vi "Weighted_Cross_Moments_raw.vi"(0 "AI Cluster 1":T5={"Colour"=0, "Inst type"=enum."Pitot-static tube", "Inst name"="Manometer voltage", "Symbol"="U", "Code name"="", "Extra Info"="U", "Inst Array"=enum."PWA", "Extra Titles"=[], "Extra Values"=[], "U"=0.0, "u^2"=0.0, "u^3"=0.0, "u^4"=0.0, "Skew_u"=0.0, "Kurt_u"=0.0, "Sd Error in Mean"=0.0, "% u'/U"=0.0, "X"=0.0, "Y"=0.0, "Z"=0.0, "Timescale integral Estimate"=0.0, "Sd Error in Variance"=0.0, "Calib File"=path "", "Calib Constants"=[], "Output Position"=FALSE, "Stats"=enum."None", "Av Sampling Rate"=0.0, "Av No of Samples"=0.0, "Total Meas Time (s)"=0.0, "ADAM Ch Name"="", "Max value"=0.0, "Min value"=0.0, "Req Sample Rate Hz"=0.0, "Sync Delay Time (s)"=0.0, "Ch No"=0, "Device"="", "Use Latest Calib"=FALSE, "Port"="", "Metadata Ch Names"=[], "Metadata Ch Values"=[], "Label"=""} {"Sync Delay Time (s)" format="%.4f"; "Total Meas Time (s)" format="%_5g"; "Sd Error in Variance" format="%_3g"; "Skew_u" format="%_3g"; "% u'/U" format="%_3g"; "Sd Error in Mean" format="%_3g"; "Kurt_u" format="%_3g"; "u^4" format="%_3g"; "u^3" format="%_3g"; "U" format="%_3g"; "u^2" format="%_3g"}, 1 "AI Cluster 2":T5={"Colour"=0, "Inst type"=enum."Pitot-static tube", "Inst name"="Manometer voltage", "Symbol"="U", "Code name"="", "Extra Info"="U", "Inst Array"=enum."PWA", "Extra Titles"=[], "Extra Values"=[], "U"=0.0, "u^2"=0.0, "u^3"=0.0, "u^4"=0.0, "Skew_u"=0.0, "Kurt_u"=0.0, "Sd Error in Mean"=0.0, "% u'/U"=0.0, "X"=0.0, "Y"=0.0, "Z"=0.0, "Timescale integral Estimate"=0.0, "Sd Error in Variance"=0.0, "Calib File"=path "", "Calib Constants"=[], "Output Position"=FALSE, "Stats"=enum."None", "Av Sampling Rate"=0.0, "Av No of Samples"=0.0, "Total Meas Time (s)"=0.0, "ADAM Ch Name"="", "Max value"=0.0, "Min value"=0.0, "Req Sample Rate Hz"=0.0, "Sync Delay Time (s)"=0.0, "Ch No"=0, "Device"="", "Use Latest Calib"=FALSE, "Port"="", "Metadata Ch Names"=[], "Metadata Ch Values"=[], "Label"=""} {"Sync Delay Time (s)" format="%.4f"; "Total Meas Time (s)" format="%_5g"; "Sd Error in Variance" format="%_3g"; "Skew_u" format="%_3g"; "% u'/U" format="%_3g"; "Sd Error in Mean" format="%_3g"; "Kurt_u" format="%_3g"; "u^4" format="%_3g"; "u^3" format="%_3g"; "U" format="%_3g"; "u^2" format="%_3g"}, 2 "Time Cluster 1":T3, 3 "Time Cluster 2":T3, 5 "Shift Cluster In":T2 {"Cross Correlation" format="%.2f"; "Stats" format="%.2f"}, 7 "Shift Input":T1, 9 "interp. method":enum16{"nearest", "linear"}(ring)=enum."linear", 10 "Time (s) 1":dbl[](array[numeric]), 11 "Time (s) 2":dbl[](array[numeric])) -> (13 "Shift Output":T1, 17 "output cluster":T4 {"Time Window (ms)" format="%.2f"; "w^2 Paired" format="%.2f"; "u^2 Paired" format="%.2f"; "u^2w^2" format="%.2f"; "u^3w" format="%.2f"; "uw^3" format="%.2f"; "uw/u'w'" format="%.2f"; "uw^2" format="%.2f"; "u^2w" format="%.2f"; "uw" format="%.2f"}, 19 "Shift Cluster Out":T2 {"Cross Correlation" format="%.2f"; "Stats" format="%.2f"})   [LabVIEW 2021]
uses:
  Controls/Analysis_info_cluster.ctl
  Controls/Inst_type.ctl
  Controls/Instrument_Array.ctl
  Controls/Correlation_cluster1.ctl
  Controls/Time_Trace_Cluster.ctl
  Controls/Cross_Moments_Shift_Cluster.ctl
  Controls/Shift_Cluster.ctl
  <vilib>/Analysis/baseanly.llb/Mean (DBL).vi
  Globals/Meas_global.vi
  <vilib>/Analysis/NI_AALBase.lvlib
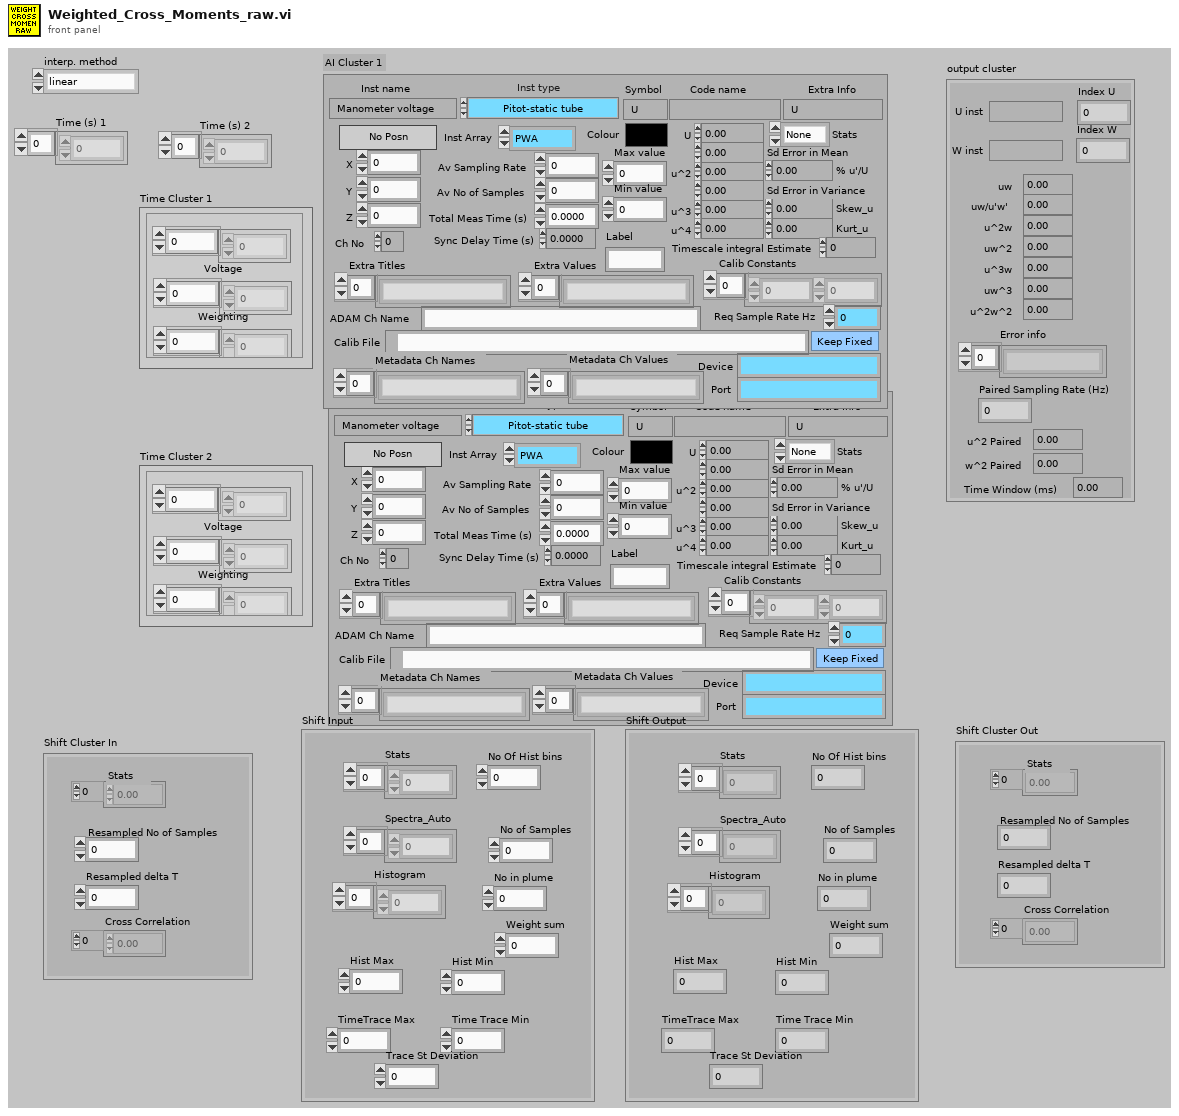
[diagram p1: front panel]
types:
  T1 = typedef "Shift_Cluster.ctl" = cluster{"Stats":dbl[], "Spectra_Auto":dbl[], "Histogram":dbl[], "Hist Max":dbl, "Hist Min":dbl, "No of Samples":i32, "No in plume":i32, "Weight sum":dbl, "No Of Hist bins":i32, "TimeTrace Max":dbl, "Time Trace Min":dbl, "Trace St Deviation":dbl}
  T2 = typedef "Cross_Moments_Shift_Cluster.ctl" = cluster{"Stats":dbl[], "Resampled No of Samples":i32, "Resampled delta T":dbl, "Cross Correlation":dbl[]}
  T3 = typedef "Time_Trace_Cluster.ctl" = cluster{"Weighting":dbl[], "Voltage":dbl[], "Eng Values":dbl[]}
  T4 = typedef "Correlation_cluster1.ctl" = cluster{"U inst":string, "uw":dbl, "u^2w":dbl, "uw^2":dbl, "uw/u'w'":dbl, "W inst":string, "uw^3":dbl, "u^3w":dbl, "u^2w^2":dbl, "Index U":i32, "Index W":i32, "Error info":string[], "Paired Sampling Rate (Hz)":dbl, "u^2 Paired":dbl, "w^2 Paired":dbl, "Time Window (ms)":dbl}
  T5 = typedef "Analysis_info_cluster.ctl" = cluster{"Colour":u32, "Inst type":T6, "Inst name":string, "Symbol":string, "Code name":string, "Extra Info":string, "Inst Array":T7, "Extra Titles":string[], "Extra Values":string[], "U":dbl, "u^2":dbl, "u^3":dbl, "u^4":dbl, "Skew_u":dbl, "Kurt_u":dbl, "Sd Error in Mean":dbl, "% u'/U":dbl, "X":dbl, "Y":dbl, "Z":dbl, "Timescale integral Estimate":dbl, "Sd Error in Variance":dbl, "Calib File":path, "Calib Constants":dbl[], "Output Position":bool, "Stats":enum16{"None", "Basic", "Full"}, "Av Sampling Rate":dbl, "Av No of Samples":dbl, "Total Meas Time (s)":dbl, "ADAM Ch Name":string, "Max value":dbl, "Min value":dbl, "Req Sample Rate Hz":dbl, "Sync Delay Time (s)":dbl, "Ch No":i16, "Device":string, "Use Latest Calib":bool, "Port":string, "Metadata Ch Names":string[], "Metadata Ch Values":string[], "Label":string}
  T6 = typedef "Inst_type.ctl" = enum16{"Raw voltage", "Raw with zero offsetting", "Propeller anemometer", "Pressure Transducer", "Pitot-static tube", "Hot wire", "Cross wire 1", "Cross wire 2", "Generic Linear", "Generic Polynomial", "Generic BackPoly", "Fast FID", "Thermocouple", "Cold wire", "Pulsed Wire", "LDA Vel", "LDA Tran time", "LDA Arr time", "Microphone"}
  T7 = typedef "Instrument_Array.ctl" = enum16{"PWA", "LDA", "Analogue"}
  T8 = typedef "Resample mode.ctl" = cluster{"Mode":enum16{"Index", "Interpolate"}, "Index":dbl[]}
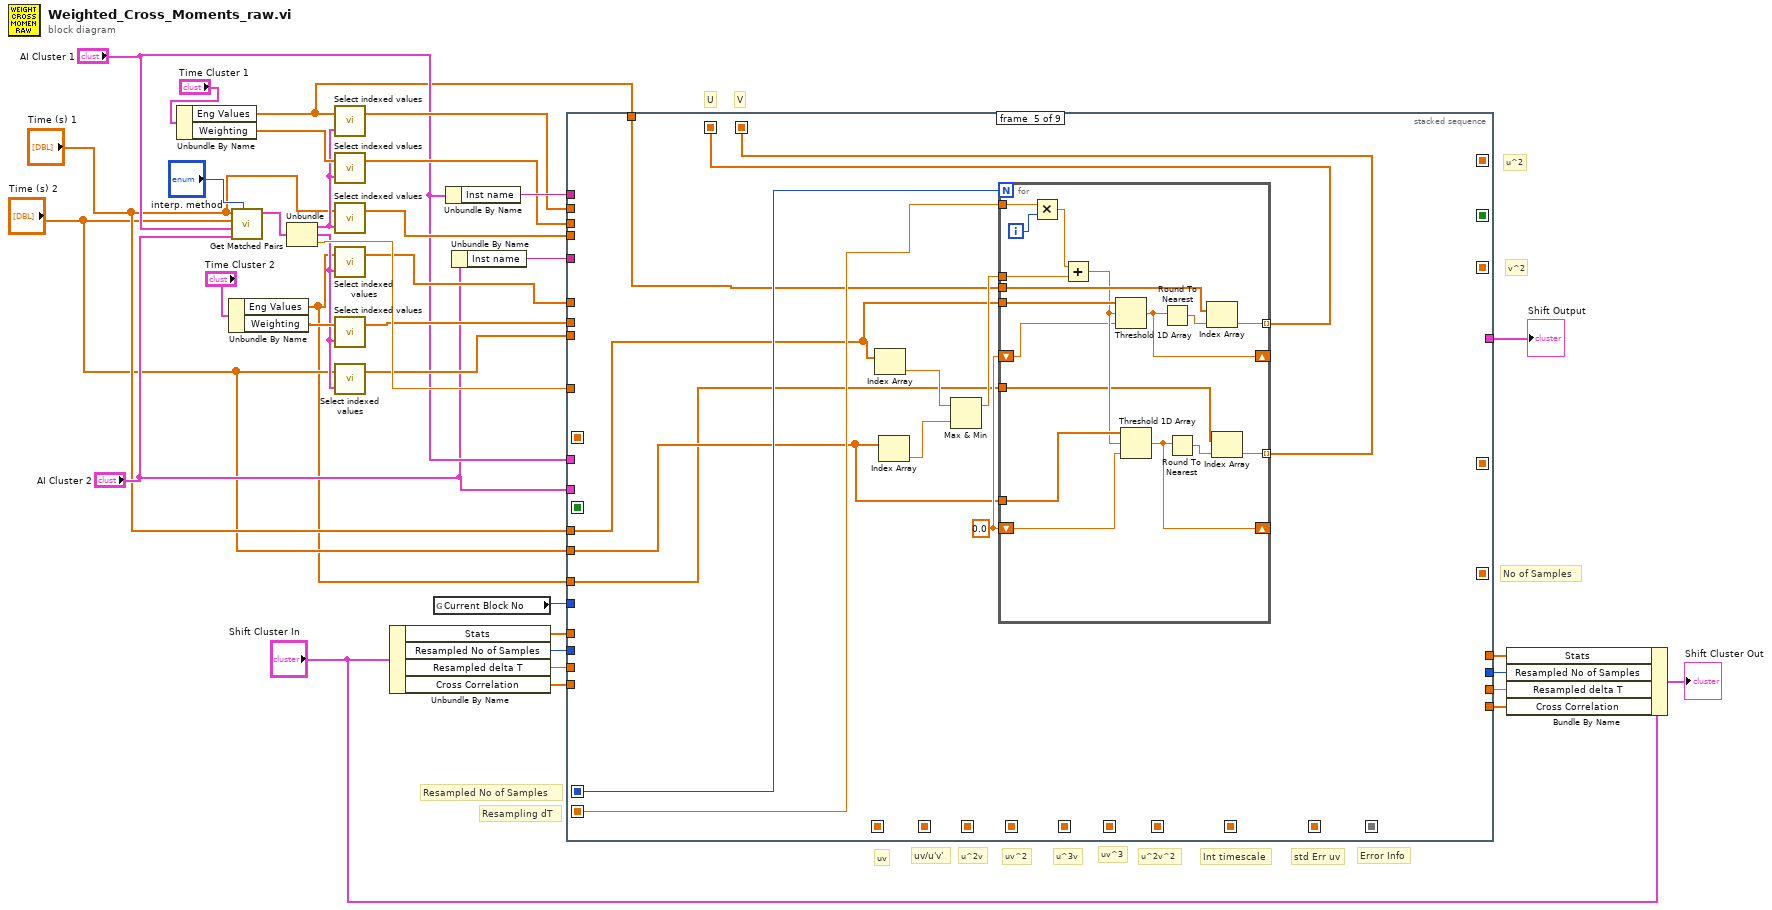
[diagram p0: block diagram]
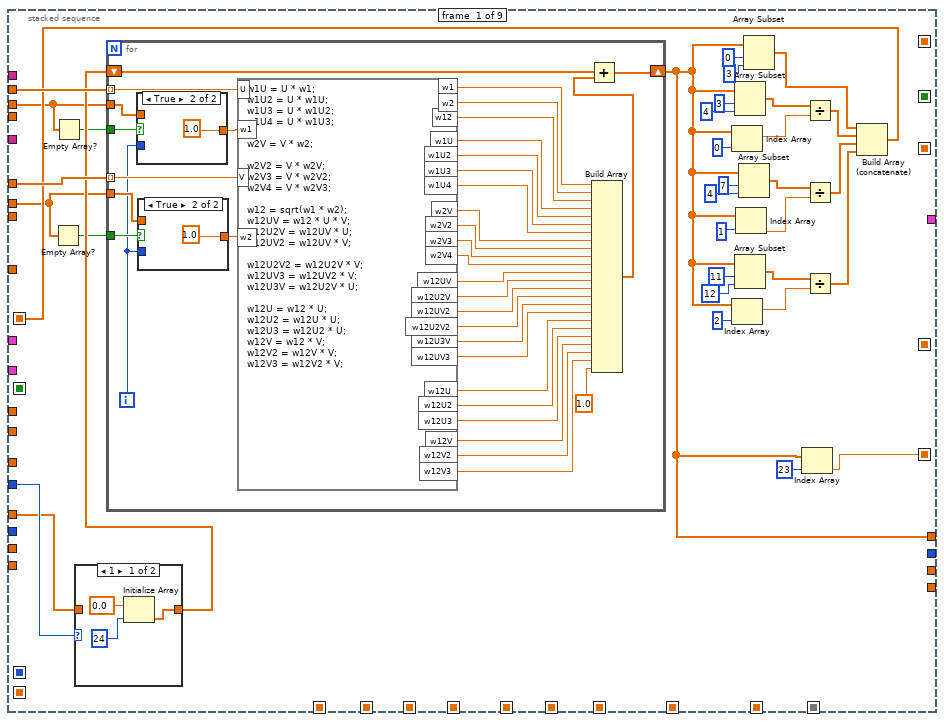
[diagram p2: hidden frame]
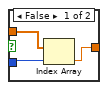
[diagram p4: hidden frame]
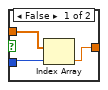
[diagram p5: hidden frame]
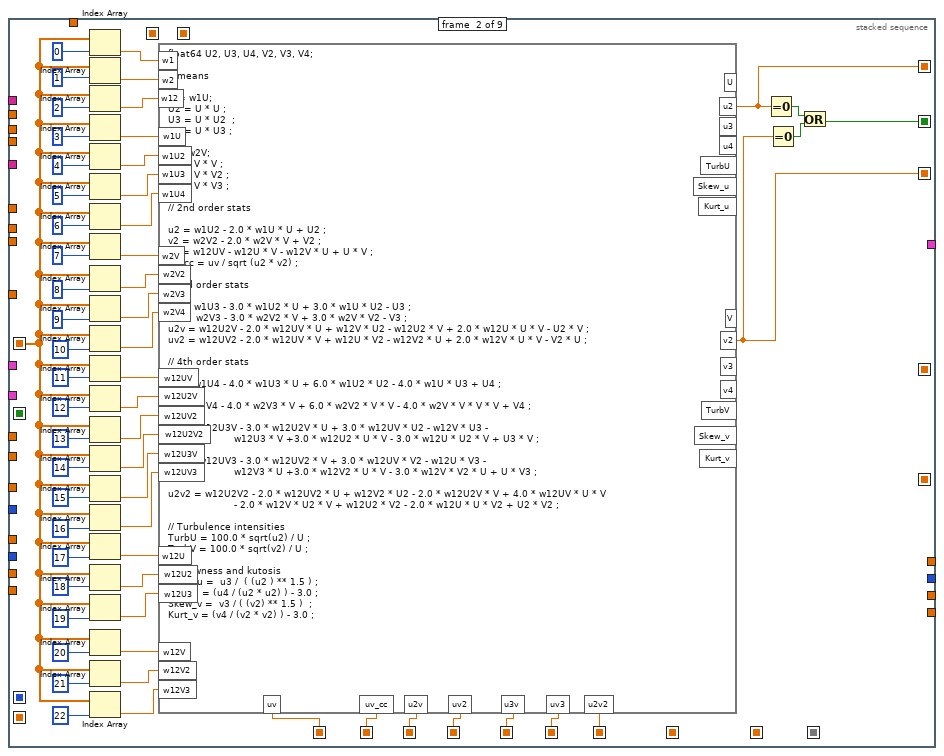
[diagram p6: hidden frame]
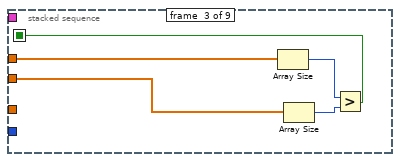
[diagram p7: hidden frame]
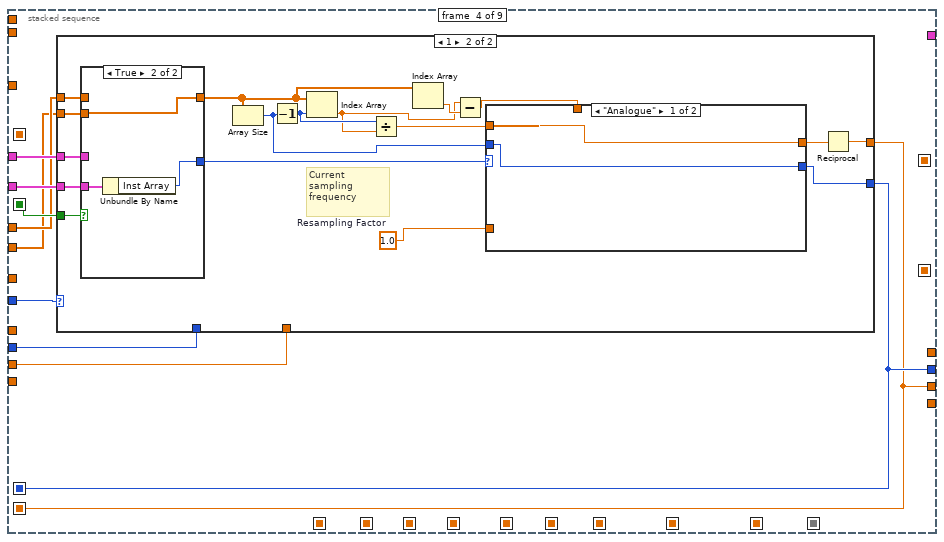
[diagram p8: hidden frame]
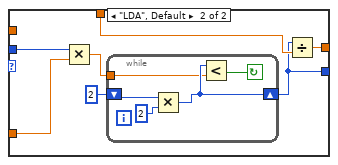
[diagram p10: hidden frame]
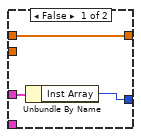
[diagram p11: hidden frame]
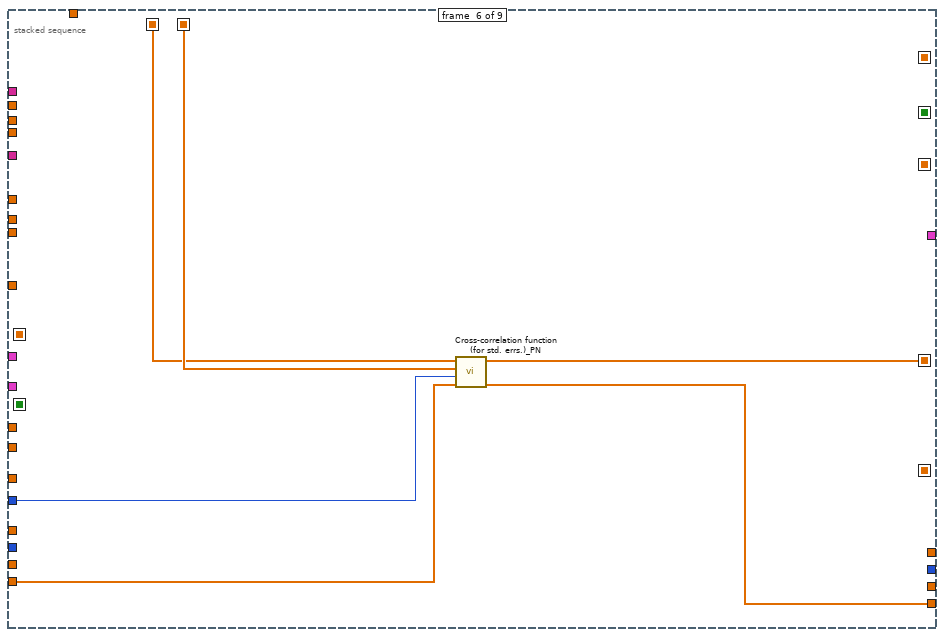
[diagram p12: hidden frame]
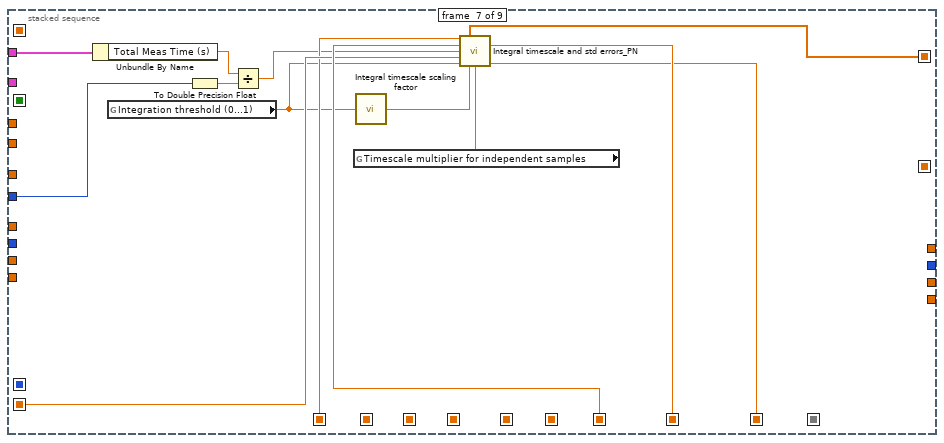
[diagram p13: hidden frame]
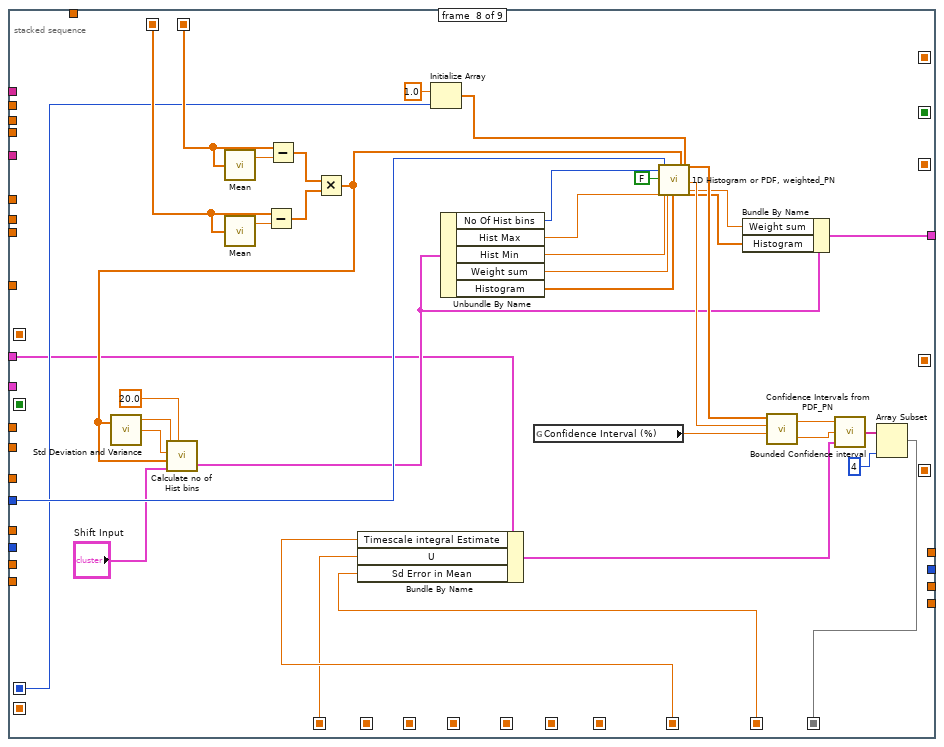
[diagram p14: hidden frame]
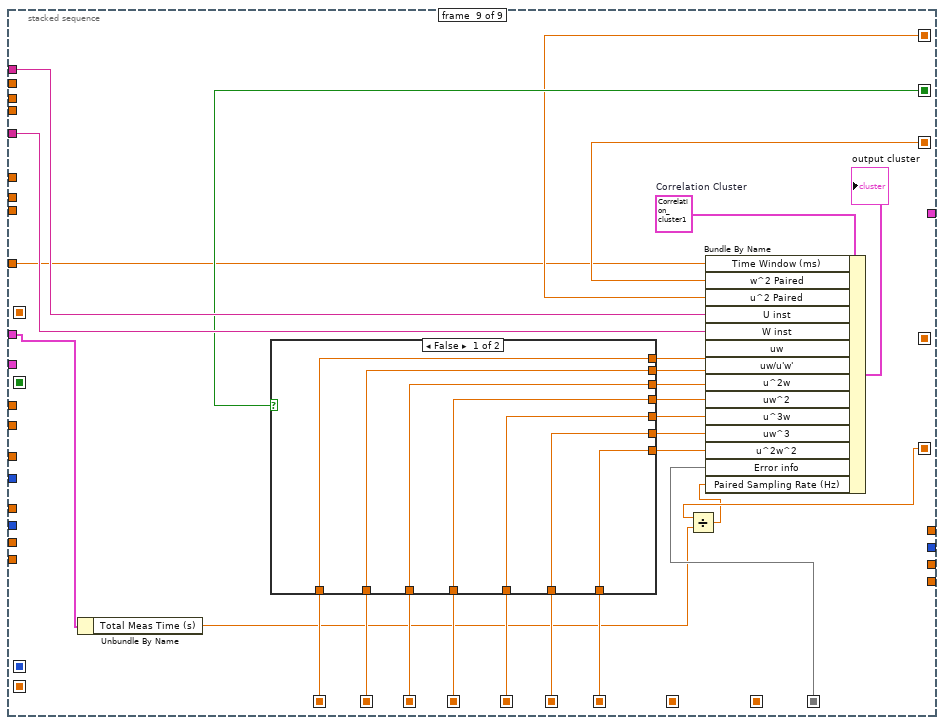
[diagram p15: hidden frame]
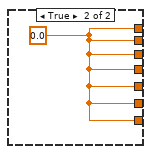
[diagram p16: hidden frame]
diagram:
  # "v^2"
  # "u^2"
  # "No of Samples"
  # "Error Info"
  # "Int timescale"
  # "std Err uv"
  # "V"
  # "U"
  # "Resampling dT"
  # "Resampled No of Samples"
  # "u^2v^2"
  # "uv^3"
  # "u^3v"
  # "uv^2"
  # "u^2v"
  # "uv/u'v'"
  # "uv"
  n1 = Unbundle By Name("Time Cluster 1") -> ("Eng Values"=w2:dbl[], "Weighting"=w20:dbl[])
  n2 = Unbundle By Name("Time Cluster 2") -> ("Eng Values"=w1:dbl[], "Weighting"=w21:dbl[])
  n3 = call "Get Matched Pairs.vi"("interp. method"="interp. method", "Cluster 2"="AI Cluster 2", "Cluster 1"="AI Cluster 1", "Time (s) 2"="Time (s) 2", "Time (s) 1"="Time (s) 1") -> ("Cluster out"=w8:cluster{"Cluster":T8, "Cluster":T8, dbl})  [unwired: 5 in, 1 out]
  n4 = Unbundle(w8) -> ("Cluster"=w9:T8, "Cluster"=w10:T8, w15:dbl)
  n5 = call "Select indexed values.vi"("Cluster"=w9, "Values"=w2) -> ("Values Out"=w16:dbl[])  [unwired: 1 in]
  n6 = call "Select indexed values.vi"("Cluster"=w9, "Values"=w20) -> ("Values Out"=w17:dbl[])  [unwired: 1 in]
  n7 = call "Select indexed values.vi"("Cluster"=w9, "Values"="Time (s) 1") -> ("Values Out"=w12:dbl[])  [unwired: 1 in]
  n8 = call "Select indexed values.vi"("Cluster"=w10, "Values"=w1) -> ("Values Out"=w14:dbl[])  [unwired: 1 in]
  n9 = call "Select indexed values.vi"("Cluster"=w10, "Values"=w21) -> ("Values Out"=w13:dbl[])  [unwired: 1 in]
  n10 = call "Select indexed values.vi"("Cluster"=w10, "Values"="Time (s) 2") -> ("Values Out"=w11:dbl[])  [unwired: 1 in]
  n11 = Unbundle By Name("Shift Cluster In") -> ("Stats"=w30:dbl[], "Resampled No of Samples"=w27:i32, "Resampled delta T"=w28:dbl, "Cross Correlation"=w24:dbl[])
  n12 = global read "Meas_global.vi" "Current Block No"() -> (w33:i32)
  n13 = Unbundle By Name("AI Cluster 1") -> ("Inst name"=w35:string)
  n14 = Unbundle By Name("AI Cluster 2") -> ("Inst name"=w34:string)
  n15 = stacked-sequence {
    seq-local: [_ w164 _ _ _ _ _ _ _] -> [_ _ _ _ _ _ w274 w290 w338]
    seq-local: [_ w163 _ _ _ _ _ _ _] -> [_ _ _ _ _ _ _ _ w337]
    seq-local: [w65 _ _ _ _ _ _ _ _] -> [_ w125 _ _ _ _ _ _ _]
    seq-local: [_ w158 _ _ _ _ _ _ _] -> [_ _ _ _ _ _ _ _ w334]
    seq-local: [_ w157 _ _ _ _ _ _ _] -> [_ _ _ _ _ _ _ _ w333]
    seq-local: [_ w138 _ _ _ _ _ _ _] -> [_ _ _ _ _ _ _ _ w331]
    seq-local: [_ w137 _ _ _ _ _ _ _] -> [_ _ _ _ _ _ _ _ w329]
    seq-local: [_ w136 _ _ _ _ _ _ _] -> [_ _ _ _ _ _ w278 _ w327]
    seq-local: [_ _ w179 _ _ _ _ _ _] -> [_ _ _ w191 _ _ _ _ _]
    seq-local: [_ _ _ w185 _ _ _ _ _] -> [_ _ _ _ w242 _ _ w305 _]
    seq-local: [_ _ _ w184 _ _ _ _ _] -> [_ _ _ _ w241 _ w277 _ _]
    seq-local: [_ _ _ _ w237 _ _ _ _] -> [_ _ _ _ _ w263 _ w312 _]
    seq-local: [_ _ _ _ w235 _ _ _ _] -> [_ _ _ _ _ w264 _ w313 _]
    seq-local: [_ _ _ _ _ w265 _ _ _] -> [_ _ _ _ _ _ w279 _ _]
    seq-local: [_ _ _ _ _ _ w273 _ _] -> [_ _ _ _ _ _ _ w289 _]
    seq-local: [_ _ _ _ _ _ w276 _ _] -> [_ _ _ _ _ _ _ w291 _]
    seq-local: [_ _ _ _ _ _ _ w282 _] -> [_ _ _ _ _ _ _ _ w340]
    seq-local: [_ w120 _ _ _ _ _ _ _] -> [_ _ _ _ _ _ _ _ w325]
    seq-local: [w40 _ _ _ _ _ _ _ _] -> [_ _ _ _ _ _ _ _ w323]
    seq-local: [_ w119 _ _ _ _ _ _ _] -> [_ _ _ _ _ _ _ _ w320]
    seq-local: [_ w118 _ _ _ _ _ _ _] -> [_ _ _ _ _ _ _ _ w319]
    tunnel: w16 -> [w69 _ _ _ _ _ _ _ _]
    tunnel: w14 -> [w68 _ _ _ _ _ _ _ _]
    tunnel: w33 -> [w67 _ _ w188 _ w262 w268 w309 _]
    tunnel: w17 -> [w39 _ _ _ _ _ _ _ _]
    tunnel: w13 -> [w38 _ _ _ _ _ _ _ _]
    tunnel: w35 -> [_ _ _ _ _ _ _ _ w343]
    tunnel: w34 -> [_ _ _ _ _ _ _ _ w342]
    tunnel: "AI Cluster 1" -> [_ _ _ w190 _ _ w275 w286 w324]
    tunnel: "AI Cluster 2" -> [_ _ _ w189 _ _ _ _ _]
    tunnel: w30 -> [w43 _ _ _ _ _ _ _ _]
    tunnel: [w41 _ _ _ _ _ _ _ _] -> w29
    tunnel: w28 -> [_ _ _ w187 _ _ _ _ _]
    tunnel: w27 -> [_ _ _ w186 _ _ _ _ _]
    tunnel: [_ _ _ w185 _ _ _ _ _] -> w26
    tunnel: [_ _ _ w184 _ _ _ _ _] -> w25
    tunnel: w24 -> [_ _ _ _ _ w261 _ _ _]
    tunnel: [_ _ _ _ _ w260 _ _ _] -> w23
    tunnel: [_ _ _ _ _ _ _ w298 _] -> w22
    tunnel: w15 -> [_ _ _ _ _ _ _ _ w318]
    tunnel: w12 -> [_ _ _ _ _ _ _ _ _]
    tunnel: w11 -> [_ _ _ _ _ _ _ _ _]
    tunnel: "Time (s) 1" -> [_ _ w178 w183 w233 _ _ _ _]
    tunnel: "Time (s) 2" -> [_ _ w177 w182 w234 _ _ _ _]
    tunnel: w2 -> [_ _ _ _ w232 _ _ _ _]
    tunnel: w1 -> [_ _ _ _ w231 _ _ _ _]
    frame #0 {
      n16 = Empty Array?(array=w38) -> (empty?=w36:bool)
      n17 = Empty Array?(array=w39) -> (empty?=w37:bool)
      n18 = case shown="1" w67 {
        tunnel: [w71 w73] -> w66
        tunnel: w43 -> [_ w73]
        frame 1 {
          n19 = Initialize Array(0.0 ("Element Data"), 24 ("Dimension Size")) -> (w71:dbl[])
        }
        frame 2, Default {
        }
      }
      n20 = for {
        shift-right: [w105] -> w41
        shift-left: w66 -> [w109]
        tunnel: w39 -> [w79]
        tunnel: w69 -> [w107] mode=indexing
        tunnel: w68 -> [w106] mode=indexing
        tunnel: w38 -> [w77]
        tunnel: w37 -> [w80]
        tunnel: w36 -> [w76]
        i -> [w75]
        n21 = case shown="True" w80 {
          tunnel: [w116 1.0] -> w78
          tunnel: w75 -> [w115 _]
          tunnel: w79 -> [w114 _]
          frame False {
            n22 = Index Array(array=w114, index=w115) -> (element=w116:dbl)
          }
          frame True {
          }
        }
        n23 = case shown="True" w76 {
          tunnel: [w112 1.0] -> w74
          tunnel: w75 -> [w111 _]
          tunnel: w77 -> [w110 _]
          frame False {
            n24 = Index Array(array=w110, index=w111) -> (element=w112:dbl)
          }
          frame True {
          }
        }
        n25 = formula code="w1U = U * w1;\nw1U2 = U * w1U;\nw1U3 = U * w1U2;\nw1U4 = U * w1U3;\n\nw2V = V * w2;\n\nw2V2 = V * w2V;\nw2V3 = V * w2V2;\nw2V4 = V * w2V3;\n\nw12 = sqrt(w1 * w2);\nw12UV = w12 * U * V;\nw12U2V = w12UV * U;\nw12UV2 = w12UV * V;\n\nw12U2V2 = w12U2V * V;\nw12UV3 = w12UV2 * V;\nw12U3V = w12U2V * U;\n\nw12U = w12 * U;\nw12U2 = w12U * U;\nw12U3 = w12U2 * U;\nw12V = w12 * V;\nw12V2 = w12V * V;\nw12V3 = w12V2 * V;"("V"=w106, "U"=w107, "w1"=w78, "w2"=w74) -> ("w12UV"=w96:dbl, "w1U"=w104:dbl, "w2V"=w100:dbl, "w1U2"=w103:dbl, "w2V2"=w99:dbl, "w12U2V"=w95:dbl, "w12UV2"=w94:dbl, "w1U3"=w102:dbl, "w1U4"=w101:dbl, "w2V3"=w98:dbl, "w2V4"=w97:dbl, "w12U3V"=w92:dbl, "w12UV3"=w91:dbl, "w12U2V2"=w93:dbl, "w12U"=w87:dbl, "w12U2"=w86:dbl, "w12U3"=w85:dbl, "w12V"=w84:dbl, "w12V2"=w83:dbl, "w12V3"=w82:dbl, "w12"=w90:dbl, "w1"=w89:dbl, "w2"=w88:dbl)
        n26 = Build Array(w89, w88, w90, w104, w103, w102, w101, w100, w99, w98, w97, w96, w95, w94, w93, w92, w91, w87, w86, w85, w84, w83, w82, 1.0) -> (w108:dbl[])
        n27 = Add(x=w109, y=w108) -> (x+y=w105:dbl[])
      }
      n28 = Index Array(array=w41, index=0 ("Index")) -> (element=w61:dbl)
      n29 = Index Array(array=w41, index=2 ("Index")) -> (element=w51:dbl)
      n30 = Array Subset(array=w41, index=3 ("Array Index"), length=4) -> (w62:dbl[])
      n31 = Array Subset(array=w41, index=11 ("Array Index"), length=12) -> (w52:dbl[])
      n32 = Index Array(array=w41, index=1 ("Index")) -> (element=w58:dbl)
      n33 = Array Subset(array=w41, index=7 ("Array Index"), length=4) -> (w57:dbl[])
      n34 = Array Subset(array=w41, index=0, length=3) -> (w44:dbl[])
      n35 = Index Array(array=w41, index=23 ("Index")) -> (element=w40:dbl)
      n36 = Divide(x=w62, y=w61) -> (x/y=w49:dbl[])
      n37 = Divide(x=w57, y=w58) -> (x/y=w48:dbl[])
      n38 = Divide(x=w52, y=w51) -> (x/y=w47:dbl[])
      n39 = Build Array (concatenate)(w44, w49, w48, w47) -> (w65:dbl[])
    }
    frame #1 {
      n40 = Index Array(array=w125, index=0) -> (element=w170:dbl)
      n41 = Index Array(array=w125, index=1) -> (element=w169:dbl)
      n42 = Index Array(array=w125, index=2) -> (element=w168:dbl)
      n43 = Index Array(array=w125, index=3) -> (element=w167:dbl)
      n44 = Index Array(array=w125, index=4) -> (element=w166:dbl)
      n45 = Index Array(array=w125, index=5) -> (element=w165:dbl)
      n46 = Index Array(array=w125, index=6) -> (element=w160:dbl)
      n47 = Index Array(array=w125, index=7) -> (element=w159:dbl)
      n48 = Index Array(array=w125, index=8) -> (element=w150:dbl)
      n49 = Index Array(array=w125, index=9) -> (element=w149:dbl)
      n50 = Index Array(array=w125, index=10) -> (element=w152:dbl)
      n51 = Index Array(array=w125, index=11) -> (element=w151:dbl)
      n52 = Index Array(array=w125, index=12) -> (element=w146:dbl)
      n53 = Index Array(array=w125, index=13) -> (element=w145:dbl)
      n54 = Index Array(array=w125, index=14) -> (element=w141:dbl)
      n55 = Index Array(array=w125, index=15) -> (element=w140:dbl)
      n56 = Index Array(array=w125, index=16) -> (element=w139:dbl)
      n57 = Index Array(array=w125, index=17) -> (element=w131:dbl)
      n58 = Index Array(array=w125, index=18) -> (element=w130:dbl)
      n59 = Index Array(array=w125, index=19) -> (element=w129:dbl)
      n60 = Index Array(array=w125, index=20) -> (element=w128:dbl)
      n61 = Index Array(array=w125, index=21) -> (element=w124:dbl)
      n62 = Index Array(array=w125, index=22) -> (element=w123:dbl)
      n63 = formula code="float64 U2, U3, U4, V2, V3, V4;\n\n// means\n\nU = w1U;\nU2 = U * U ;\nU3 = U * U2  ;\nU4 = U * U3 ;\n\nV = w2V;\nV2 = V * V ;\nV3 = V * V2 ;\nV4 = V * V3 ;\n\n// 2nd order stats\n\nu2 = w1U2 - 2.0 * w1U * U + U2 ;\nv2 = w2V2 - 2.0 * w2V * V + V2 ;\nuv = w12UV - w12U * V - w12V * U + U * V ;\nuv_cc = uv / sqrt (u2 * v2) ;\n\n// 3rd order stats\n\nu3 = w1U3 - 3.0 * w1U2 * U + 3.0 * w1U * U2 - U3 ;\nv3 =  w2V3 - 3.0 * w2V2 * V + 3.0 * w2V * V2 - V3 ;\nu2v = w12U2V - 2.0 * w12UV * U + w12V * U2 - w12U2 * V + 2.0 * w12U * U * V - U2 * V ;\nuv2 = w12UV2 - 2.0 * w12UV * V + w12U * V2 - w12V2 * U + 2.0 * w12V * U * V - V2 * U ;\n\n// 4th order stats\n\nu4 = w1U4 - 4.0 * w1U3 * U + 6.0 * w1U2 * U2 - 4.0 * w1U * U3 + U4 ;\n\nv4 = w2V4 - 4.0 * w2V3 * V + 6.0 * w2V2 * V * V - 4.0 * w2V * V * V * V + V4 ;\n\nu3v = w12U3V - 3.0 * w12U2V * U + 3.0 * w12UV * U2 - w12V * U3 - \n                      w12U3 * V +3.0 * w12U2 * U * V - 3.0 * w12U * U2 * V + U3 * V ;\n\nuv3 = w12UV3 - 3.0 * w12UV2 * V + 3.0 * w12UV * V2 - w12U * V3 - \n                      w12V3 * U +3.0 * w12V2 * U * V - 3.0 * w12V * V2 * U + U * V3 ;\n\nu2v2 = w12U2V2 - 2.0 * w12UV2 * U + w12V2 * U2 - 2.0 * w12U2V * V + 4.0 * w12UV * U * V\n                      - 2.0 * w12V * U2 * V + w12U2 * V2 - 2.0 * w12U * U * V2 + U2 * V2 ; \n\n// Turbulence intensities\nTurbU = 100.0 * sqrt(u2) / U ;\nTurbV = 100.0 * sqrt(v2) / U ;\n\n// Skewness and kutosis\nSkew_u =  u3 /  ( (u2 ) ** 1.5 ) ;\nKurt_u = (u4 / (u2 * u2) ) - 3.0 ;\nSkew_v =  v3 / ( (v2) ** 1.5 )  ;\nKurt_v = (v4 / (v2 * v2) ) - 3.0 ;"("w1"=w170, "w2"=w169, "w12"=w168, "w1U2"=w166, "w1U3"=w165, "w1U"=w167, "w1U4"=w160, "w2V"=w159, "w2V2"=w150, "w2V4"=w152, "w2V3"=w149, "w12UV"=w151, "w12U2V"=w146, "w12UV2"=w145, "w12U2V2"=w141, "w12U3V"=w140, "w12UV3"=w139, "w12U2"=w130, "w12U3"=w129, "w12V"=w128, "w12V2"=w124, "w12U"=w131, "w12V3"=w123) -> ("uv"=w164:dbl, "u2"=w119:dbl, "v2"=w118:dbl, "uv_cc"=w163:dbl, "u2v"=w158:dbl, "uv2"=w157:dbl, "u3v"=w138:dbl, "uv3"=w137:dbl, "u2v2"=w136:dbl)  [unwired: 12 out]
      n64 = Equal To 0?(x=w119) -> (x = 0?=w122:bool)
      n65 = Equal To 0?(x=w118) -> (x = 0?=w121:bool)
      n66 = Or(x=w122, y=w121) -> (x .or. y?=w120:bool)
    }
    frame #2 {
      n67 = Array Size(array=w178) -> (size(s)=w181:i32)
      n68 = Array Size(array=w177) -> (size(s)=w180:i32)
      n69 = Greater?(x=w181, y=w180) -> (0:w179:bool)
    }
    frame #3 {
      n70 = case shown="1" w188 {
        tunnel: w191 -> [_ w210]
        tunnel: w182 -> [_ w209]
        tunnel: w190 -> [_ w207]
        tunnel: w189 -> [_ w206]
        tunnel: [w192 w204] -> w185
        tunnel: [w193 w195] -> w184
        tunnel: w187 -> [w193 _]
        tunnel: w186 -> [w192 _]
        tunnel: w183 -> [_ w194]
        frame Default {
        }
        frame 1 {
          w200 = 1.0  # Resampling Factor
          # "Current sampling\nfrequency"
          n71 = case shown="True" w210 {
            tunnel: w209 -> [_ w228]
            tunnel: [w225 w228] -> w208
            tunnel: w207 -> [w227 _]
            tunnel: w206 -> [_ w230]
            tunnel: [w226 w229] -> w205
            tunnel: w194 -> [w225 _]
            frame False {
              n72 = Unbundle By Name(w227) -> ("Inst Array"=w226:T7)
            }
            frame True {
              n73 = Unbundle By Name(w230) -> ("Inst Array"=w229:T7)
            }
          }
          n74 = Array Size(array=w208) -> (size(s)=w201:i32)
          n75 = Decrement(x=w201) -> (x-1=w202:i32)
          n76 = Index Array(array=w208, index=w202) -> (element=w197:dbl)
          n77 = Divide(x=w202, y=w197) -> (x/y=w203:dbl)
          n78 = Index Array(array=w208) -> (element=w199:dbl)  [unwired: 1 in]
          n79 = Subtract(x=w197, y=w199) -> (x-y=w198:dbl)
          n80 = case shown="\"Analogue\"" w205 {
            tunnel: w203 -> [w212 _]
            tunnel: w198 -> [_ w219]
            tunnel: [w212 w218] -> w196
            tunnel: w201 -> [w211 w216]
            tunnel: [w211 w215] -> w204
            tunnel: w200 -> [_ w214]
            frame "Analogue" {
            }
            frame "LDA", Default {
              n81 = Multiply(x=w216, y=w214) -> (x*y=w217:dbl)
              n82 = while {
                shift-right: [w222] -> w215
                shift-left: 2 -> [w224]
                tunnel: w217 -> [w220]
                stop <- w221 continue-if-true
                n83 = Multiply(x=w224, y=2) -> (x*y=w222:i32)
                n84 = Less?(x=w222, y=w220) -> (x < y?=w221:bool)
              }
              n85 = Divide(x=w215, y=w219) -> (x/y=w218:dbl)
            }
          }
          n86 = Reciprocal(x=w196) -> (1/x=w195:dbl)
        }
      }
    }
    frame #4 {
      w236 = 0.0
      n87 = Index Array(array=w233) -> (element=w240:dbl)  [unwired: 1 in]
      n88 = Index Array(array=w234) -> (element=w239:dbl)  [unwired: 1 in]
      n89 = Max & Min(x=w240, y=w239) -> (max(x,y)=w238:dbl)  [unwired: 1 out]
      n90 = for {
        N: w242 -> [_]
        tunnel: w241 -> [w259]
        tunnel: w238 -> [w256]
        tunnel: w233 -> [w255]
        tunnel: w232 -> [w253]
        tunnel: [w252] -> w237 mode=indexing
        tunnel: w234 -> [w250]
        shift-right: [w247] -> _
        shift-left: w236 -> [w248]
        shift-right: [w245] -> _
        shift-left: w236 -> [w246]
        tunnel: w231 -> [w244]
        tunnel: [w243] -> w235 mode=indexing
        i -> [w258]
        n91 = Multiply(x=w259, y=w258) -> (x*y=w257:dbl)
        n92 = Add(x=w257, y=w256) -> (x+y=w249:dbl)
        n93 = Threshold 1D Array(1:w246, 2:w249, 3:w255) -> (0:w245:dbl)
        n94 = Threshold 1D Array(1:w248, 2:w249, 3:w250) -> (0:w247:dbl)
        n95 = Round To Nearest(number=w245) -> (nearest integer value=w254:dbl)
        n96 = Round To Nearest(number=w247) -> (nearest integer value=w251:dbl)
        n97 = Index Array(array=w253, index=w254) -> (element=w252:dbl)
        n98 = Index Array(array=w244, index=w251) -> (element=w243:dbl)
      }
    }
    frame #5 {
      n99 = call "Cross-correlation function (for std. errs.)_PN.vi"("Shift in"=w261, "Current Block No"=w262, "V (m/s)"=w264, "U (m/s)"=w263) -> ("Shift Out"=w260:dbl[], "Cross-correlation function"=w265:dbl[])  [unwired: 2 in]
    }
    frame #6 {
      n100 = Unbundle By Name(w275) -> ("Total Meas Time (s)"=w271:dbl)
      n101 = global read "Meas_global.vi" "Integration threshold (0...1)"() -> (w266:dbl)
      n102 = To Double Precision Float(number=w268) -> (double precision float=w269:dbl)
      n103 = Divide(x=w271, y=w269) -> (x/y=w270:dbl)
      n104 = global read "Meas_global.vi" "Timescale multiplier for independent samples"() -> (w272:dbl)
      n105 = call "Integral timescale scaling factor.vi"("Integration threshold (0...1)"=w266) -> ("Integral timescale scaling factor"=w267:dbl)
      n106 = call "Integral timescale and std errors_PN.vi"("uv_bar (m/s)^2"=w274, "Cross-correlation function"=w279, "u2v2_bar (m/s)^4"=w278, "T_meas (s)"=w270, "dt (s)"=w277, "integral cut-off"=w266, "integral post-mult"=w267, "Timescale multiple for independent samples"=w272) -> ("Integral timescale (s)"=w276:dbl, "Std. err in uv (m/s^2)"=w273:dbl)  [unwired: 4 in, 2 out]
    }
    frame #7 {
      n107 = call-poly <vilib>:"Mean.vi"("X"=w313) -> ("mean"=w314:dbl)  [unwired: 1 out]
      n108 = call-poly <vilib>:"Mean.vi"("X"=w312) -> ("mean"=w315:dbl)  [unwired: 1 out]
      n109 = Subtract(x=w312, y=w315) -> (x-y=w317:dbl[])
      n110 = Subtract(x=w313, y=w314) -> (x-y=w316:dbl[])
      n111 = Multiply(x=w316, y=w317) -> (x*y=w303:dbl[])
      n112 = call <vilib>:"Std Deviation and Variance.vi"("X"=w303) -> ("mean"=w301:dbl, "standard deviation"=w302:dbl)  [unwired: 1 in, 1 out]
      n113 = call "Calculate no of Hist bins.vi"("Mean"=w301, "Standard Deviation"=w302, "Time Trace"=w303, "Shift Input"="Shift Input", "Number of Bins per Sigma"=20.0) -> ("Shift Output"=w299:T1)  [unwired: 1 in]
      n114 = Bundle By Name(cluster=w286, "Timescale integral Estimate"=w291, "U"=w290, "Sd Error in Mean"=w289) -> (w280:T5)
      n115 = Initialize Array(1.0, w305) -> (w310:dbl[])
      n116 = Unbundle By Name(w299) -> ("No Of Hist bins"=w294:i32, "Hist Max"=w293:dbl, "Hist Min"=w292:dbl, "Weight sum"=w295:dbl, "Histogram"=w300:dbl[])
      n117 = global read "Meas_global.vi" "Confidence Interval (%)"() -> (w285:dbl)
      n118 = call "1D Histogram or PDF, weighted_PN.vi"("Nbins"=w294, "Mean shift"=FALSE, "max"=w293, "Current block no."=w309, "min"=w292, "Shift SumW in"=w295, "Shift PDF in"=w300, "1D data"=w303, "Weights"=w310) -> ("1D histogram or PDF"=w306:dbl[], "bin width"=w307:dbl, "Shift SumW out"=w296:dbl, "Shift PDF out"=w297:dbl[])  [unwired: 14 in, 1 out]
      n119 = Bundle By Name(cluster=w299, "Weight sum"=w296, "Histogram"=w297) -> (w298:T1)
      n120 = call "Confidence Intervals from PDF_PN.vi"("Desired confidence interval (%)"=w285, "PDF bin width"=w307, "Marginal 1D PDF"=w306) -> ("Lower limit scale factor on SD or SE"=w287:dbl, "Upper limit scale factor on SD or SE"=w288:dbl)  [unwired: 1 in]
      n121 = call "Bounded Confidence interval.vi"("Analysis_info_cluster"=w280, "Lower limit scale factor on SD or SE"=w287, "Upper limit scale factor on SD or SE"=w288) -> ("Error values"=w284:string[])
      n122 = Array Subset(array=w284, length=4) -> (w282:string[])  [unwired: 1 in]
    }
    frame #8 {
      w344 = T4 {"U inst"="", "uw"=0.0, "u^2w"=0.0, "uw^2"=0.0, "uw/u'w'"=0.0, "W inst"="", "uw^3"=0.0, "u^3w"=0.0, "u^2w^2"=0.0, "Index U"=0, "Index W"=0, "Error info"=[], "Paired Sampling Rate (Hz)"=0.0, "u^2 Paired"=0.0, "w^2 Paired"=0.0, "Time Window (ms)"=0.0}  # Correlation Cluster
      n123 = Unbundle By Name(w324) -> ("Total Meas Time (s)"=w322:dbl)
      n124 = case shown="False" w325 {
        tunnel: [w351 w352] -> w339
        tunnel: w338 -> [w351 _]
        tunnel: w337 -> [w350 _]
        tunnel: [w350 w352] -> w336
        tunnel: [w349 w352] -> w335
        tunnel: w334 -> [w349 _]
        tunnel: w333 -> [w348 _]
        tunnel: [w348 w352] -> w332
        tunnel: w331 -> [w347 _]
        tunnel: [w347 w352] -> w330
        tunnel: w329 -> [w346 _]
        tunnel: [w346 w352] -> w328
        tunnel: w327 -> [w345 _]
        tunnel: [w345 w352] -> w326
        frame False {
        }
        frame True {
          w352 = 0.0 ("uv")
        }
      }
      n125 = Divide(x=w323, y=w322) -> (x/y=w321:dbl)
      n126 = Bundle By Name(cluster=w344, "Time Window (ms)"=w318, "w^2 Paired"=w319, "u^2 Paired"=w320, "U inst"=w343, "W inst"=w342, "uw"=w339, "uw/u'w'"=w336, "u^2w"=w335, "uw^2"=w332, "u^3w"=w330, "uw^3"=w328, "u^2w^2"=w326, "Error info"=w340, "Paired Sampling Rate (Hz)"=w321) -> (→"output cluster":T4)
    }
  }
  "Shift Output" <- w22
  n127 = Bundle By Name(cluster="Shift Cluster In", "Stats"=w29, "Resampled No of Samples"=w26, "Resampled delta T"=w25, "Cross Correlation"=w23) -> (→"Shift Cluster Out":T2)
